vi "A11rowmm.vi"(11 "Basic Size":dbl) -> (3 "Row":dbl)   [LabVIEW 2023]
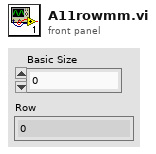
[diagram p1: front panel]
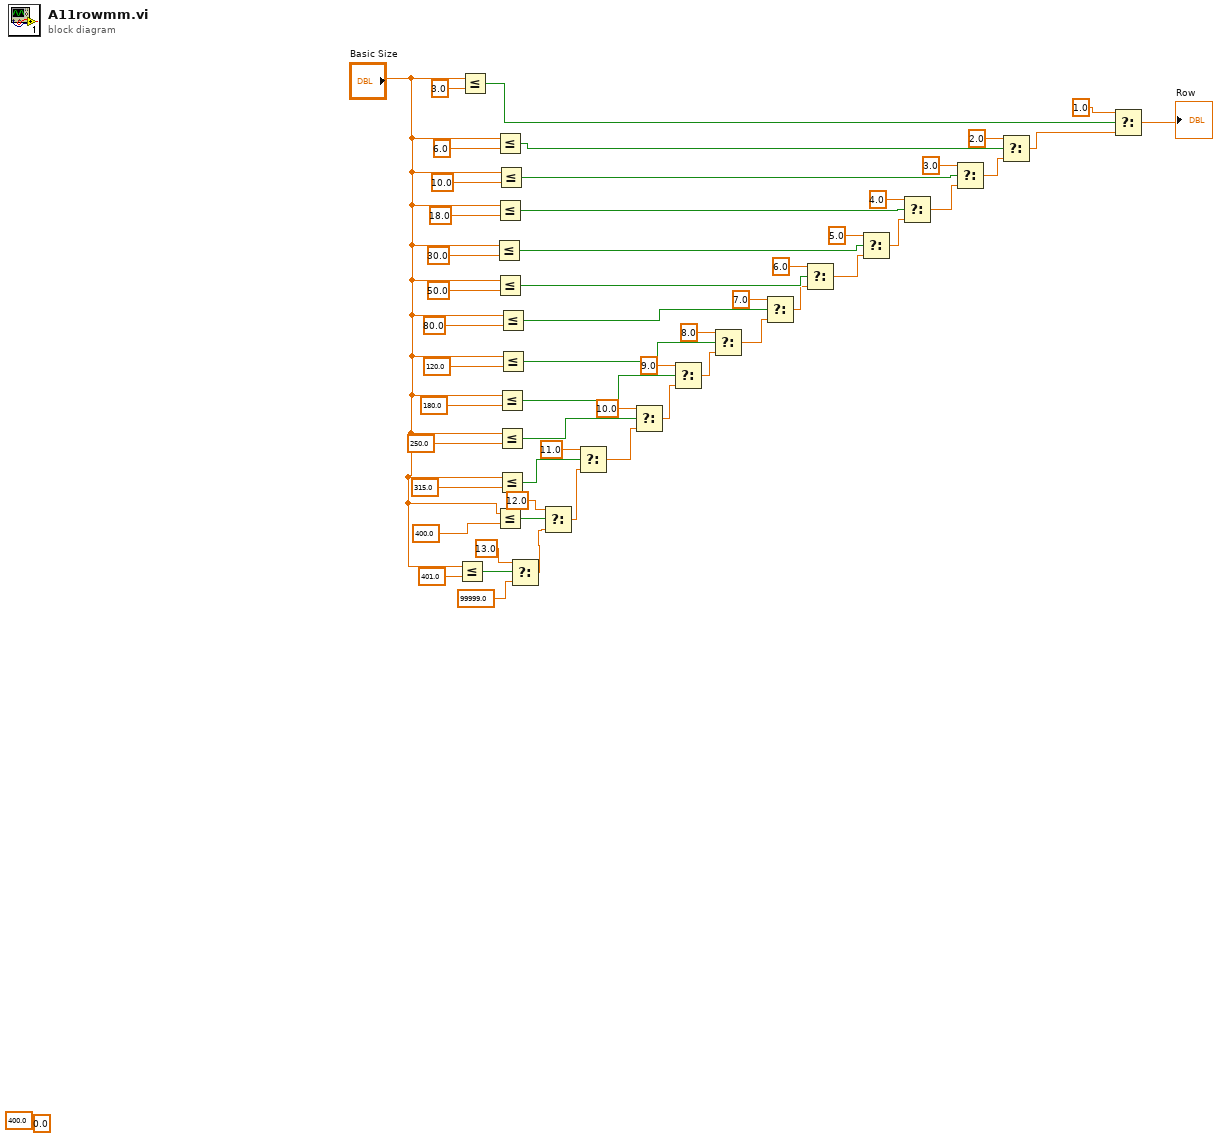
[diagram p0: block diagram]
diagram:
  (unwired) 0.0 ("f")
  (unwired) 400.0 ("y")
  n1 = Less Or Equal?(x="Basic Size", y=401.0) -> (x <= y?=w6:bool)
  n2 = Less Or Equal?(x="Basic Size", y=3.0) -> (x <= y?=w53:bool)
  n3 = Less Or Equal?(x="Basic Size", y=30.0) -> (x <= y?=w37:bool)
  n4 = Less Or Equal?(x="Basic Size", y=6.0) -> (x <= y?=w49:bool)
  n5 = Less Or Equal?(x="Basic Size", y=18.0) -> (x <= y?=w41:bool)
  n6 = Less Or Equal?(x="Basic Size", y=50.0) -> (x <= y?=w33:bool)
  n7 = Less Or Equal?(x="Basic Size", y=400.0 ("x")) -> (x <= y?=w11:bool)
  n8 = Less Or Equal?(x="Basic Size", y=10.0) -> (x <= y?=w46:bool)
  n9 = Less Or Equal?(x="Basic Size", y=180.0) -> (x <= y?=w21:bool)
  n10 = Less Or Equal?(x="Basic Size", y=250.0) -> (x <= y?=w17:bool)
  n11 = Less Or Equal?(x="Basic Size", y=315.0) -> (x <= y?=w13:bool)
  n12 = Less Or Equal?(x="Basic Size", y=80.0) -> (x <= y?=w29:bool)
  n13 = Less Or Equal?(x="Basic Size", y=120.0) -> (x <= y?=w25:bool)
  n14 = Select(t=13.0, s=w6, f=99999.0) -> (s? t:f=w5:dbl)
  n15 = Select(t=12.0, s=w11, f=w5) -> (s? t:f=w10:dbl)
  n16 = Select(t=11.0, s=w13, f=w10) -> (s? t:f=w15:dbl)
  n17 = Select(t=10.0, s=w17, f=w15) -> (s? t:f=w20:dbl)
  n18 = Select(t=9.0, s=w21, f=w20) -> (s? t:f=w23:dbl)
  n19 = Select(t=8.0, s=w25, f=w23) -> (s? t:f=w27:dbl)
  n20 = Select(t=7.0, s=w29, f=w27) -> (s? t:f=w31:dbl)
  n21 = Select(t=6.0, s=w33, f=w31) -> (s? t:f=w35:dbl)
  n22 = Select(t=5.0, s=w37, f=w35) -> (s? t:f=w39:dbl)
  n23 = Select(t=4.0, s=w41, f=w39) -> (s? t:f=w43:dbl)
  n24 = Select(t=3.0, s=w46, f=w43) -> (s? t:f=w47:dbl)
  n25 = Select(t=2.0, s=w49, f=w47) -> (s? t:f=w50:dbl)
  n26 = Select(t=1.0, s=w53, f=w50) -> (s? t:f=→"Row":dbl)
